vi "SSC Digital PPMU Configure Aperture Time.vi"(0 "Digital SSC in":T1[](array[typedef]), 5 "Aperture Time (s)":dbl format="%#_6p", 11 "error in":errorcluster) -> (4 "Digital SSC out":T1[](array[typedef]), 15 "error out":errorcluster)   [LabVIEW 2020]
doc: "Configures the aperture time for the PPMU measurement on the specified pin(s) and pin group(s)."
uses:
  SSC Digital.ctl
  <instrlib>/niDigital/niDigital.llb/niDigital PMU Aperture Time Units.ctl
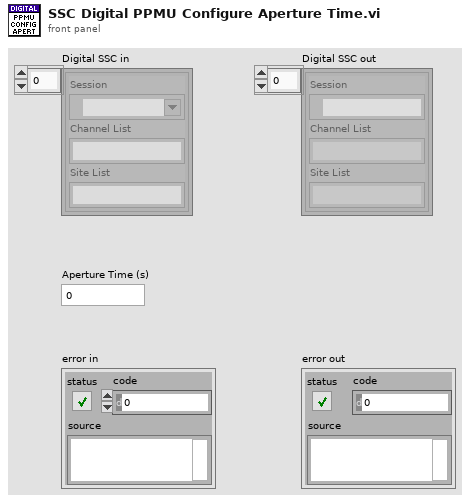
[diagram p1: front panel]
types:
  T1 = typedef "SSC Digital.ctl" = cluster{"Session":refnum<k15>, "Channel List":string, "Site List":string}
  T2 = typedef "niDigital PMU Aperture Time Units.ctl" = i32
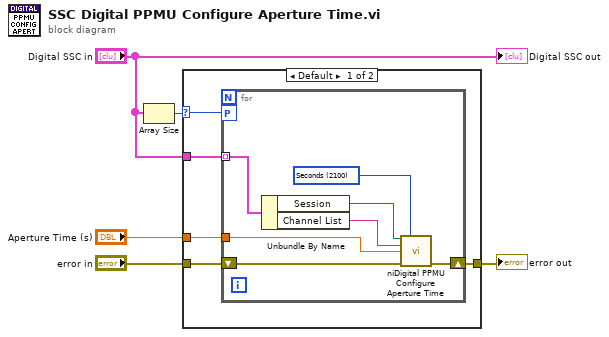
[diagram p0: block diagram]
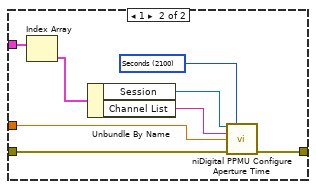
[diagram p2: hidden frame]
diagram:
  n1 = Array Size(array="Digital SSC in") -> (size(s)=w2:i32)
  n2 = case shown="Default" w2 {
    selector: w2 -> [w7 _]
    tunnel: "error in" -> [w10 w25]
    tunnel: "Aperture Time (s)" -> [w9 w24]
    tunnel: [w8 w23] -> w3
    tunnel: "Digital SSC in" -> [w6 w22]
    frame Default {
      n3 = for {
        workers-P: w7 -> [_]
        tunnel: w6 -> [w14] mode=indexing
        tunnel: w9 -> [w12]
        shift-right: [w16] -> w8
        shift-left: w10 -> [w17]
        w11 = T2 2100 items=["Seconds"=2100] ("aperture time units")
        n4 = Unbundle By Name(w14) -> ("Session"=w15:refnum<k15>, "Channel List"=w13:string)
        n5 = call <instrlib>:"niDigital PPMU Configure Aperture Time.vi"("instrument handle"=w15, "aperture time units"=w11, "channel list"=w13, "aperture time"=w12, "error in"=w17) -> ("error out"=w16:errorcluster)  [unwired: 9 in, 1 out]
      }
    }
    frame 1 {
      w19 = T2 2100 items=["Seconds"=2100] ("aperture time units")
      n6 = Index Array(array=w22) -> (element=w18:T1)  [unwired: 1 in]
      n7 = Unbundle By Name(w18) -> ("Session"=w21:refnum<k15>, "Channel List"=w20:string)
      n8 = call <instrlib>:"niDigital PPMU Configure Aperture Time.vi"("instrument handle"=w21, "aperture time units"=w19, "channel list"=w20, "aperture time"=w24, "error in"=w25) -> ("error out"=w23:errorcluster)  [unwired: 9 in, 1 out]
    }
  }
  "error out" <- w3
  "Digital SSC out" <- "Digital SSC in"
